vi "mro is Monitoring Enabled.vi"(8 "error in (no error)":errorcluster) -> (0 "error out":errorcluster, 1 "function return":i8, 2 "status out":i32)   [LabVIEW 2016, in "mirao52e_32bit.lvlib"]
doc: "MIRAOEXPORT MroBoolean MIRAOCALL mro_isMonitoringEnabled( \n MroBoolean* enabled,\n int* status\n );"
uses:
  mirao52e_32bit.lvlib
  MRO Error codes.ctl
  mirao52e.dll
panel:
  out "Monitoring enabled?":bool
  out "enabled out":i32
  out "MRO Error code":T1
  out "MRO_TRUE ?":bool
  # "Is Monitoring Enabled?"
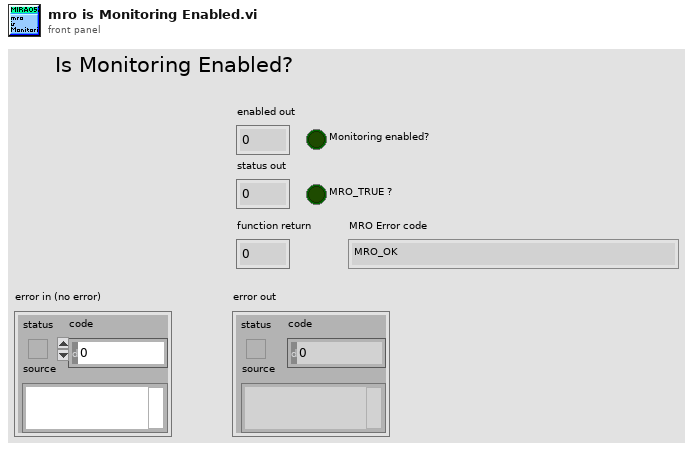
[diagram p1: front panel]
types:
  T1 = typedef "MRO Error codes.ctl" = enum16{"MRO_OK", "MRO_UNKNOWN_ERROR", "MRO_DEVICE_NOT_OPENED_ERROR", "MRO_DEFECTIVE_DEVICE_ERROR", "MRO_DEVICE_ALREADY_OPENED_ERROR", "MRO_DEVICE_IO_ERROR", "MRO_DEVICE_LOCKED_ERROR", "MRO_DEVICE_DISCONNECTED_ERROR", "MRO_DEVICE_DRIVER_ERROR", "MRO_FILE_EXISTS_ERROR", "MRO_FILE_FORMAT_ERROR", "MRO_FILE_IO_ERROR", "MRO_INVALID_COMMAND_ERROR", "MRO_NULL_POINTER_ERROR", "MRO_OUT_OF_BOUNDS_ERROR", "MRO_OPERATION_ONGOING_ERROR", "MRO_SYSTEM_ERROR", "MRO_UNAVAILABLE_DATA_ERROR", "MRO_UNDEFINED_VALUE_ERROR", "MRO_OUT_OF_SPECIFICATIONS_ERROR", "MRO_FILE_FORMAT_VERSION_ERROR", "MRO_USB_INVALID_HANDLE", "MRO_USB_DEVICE_NOT_FOUND", "MRO_USB_DEVICE_NOT_OPENED", "MRO_USB_IO_ERROR", "MRO_USB_INSUFFICIENT_RESOURCES", "MRO_USB_INVALID_BAUD_RATE", "MRO_USB_NOT_SUPPORTED", "MRO_FILE_IO_EACCES", "MRO_FILE_IO_EAGAIN", "MRO_FILE_IO_EBADF", "MRO_FILE_IO_EINVAL", "MRO_FILE_IO_EMFILE", "MRO_FILE_IO_ENOENT", "MRO_FILE_IO_ENOMEM", "MRO_FILE_IO_ENOSPC"}
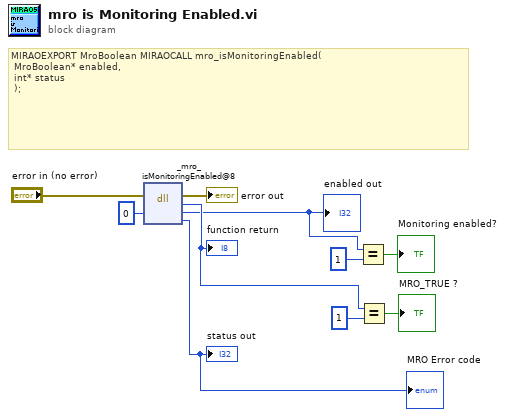
[diagram p0: block diagram]
diagram:
  # "MIRAOEXPORT MroBoolean MIRAOCALL mro_isMonitoringEnabled( \n\tMroBoolean* enabled,\n\tint* status\n\t);"
  n1 = dll-call lib="C:/Users/nvladim/Documents/Nikita-MDC/code/LabView/miraoDriver_32bit/mirao52e.*" fn="_mro_isMonitoringEnabled@8"(error in="error in (no error)", "enabled"=0) -> (error out=→"error out":errorcluster, "return type"=w6:i8, "enabled"=w1:i32, "status"=→"status out" →"MRO Error code":i32)  [unwired: 3 in, 1 out]
  "function return" <- w6
  "enabled out" <- w1
  n2 = Equal?(x=w1, y=i8 1) -> (x = y?=→"Monitoring enabled?":bool)
  n3 = Equal?(x=w6, y=i8 1) -> (x = y?=→"MRO_TRUE ?":bool)
